vi "To Camel Case.vi"   [LabVIEW 2020, in "openg_string.lvlib"]
doc: "Converts alphabetic characters in string to proper case (i.e., first alphabetic character to uppercase, all others to lowercase for each \"word,\" removing spaces between words)."
uses:
  openg_string.lvlib
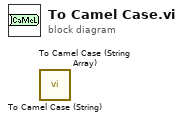
[diagram p0: block diagram]
diagram:
  n1 = call "To Camel Case (String).vi"() -> ()  [unwired: 2 in, 1 out]
  n2 = call "To Camel Case (String Array).vi"() -> ()  [unwired: 2 in, 1 out]
